vi "hmi_gun.vi"(11 "UserData":T1) -> ()   [LabVIEW 2011]
uses:
  user_data.ctl
  user_buttons_dualaction.ctl
  user_buttons_360.ctl
  gun/gun_tracking_mode.ctl
  signals/Signal.ctl
  Robot Global Data.vi
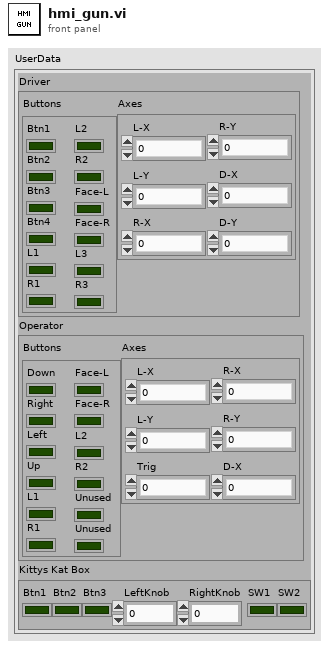
[diagram p1: front panel]
types:
  T1 = typedef "user_data.ctl" = cluster{"Driver":cluster{"Buttons":T2, "Axes":cluster{"L-X":dbl, "L-Y":dbl, "R-X":dbl, "R-Y":dbl, "D-X":dbl, "D-Y":dbl}}, "Operator":cluster{"Buttons":T3, "Axes":cluster{"L-X":dbl, "L-Y":dbl, "Trig":dbl, "R-X":dbl, "R-Y":dbl, "D-X":dbl}}, "Kittys Kat Box":cluster{"Btn1":bool, "Btn2":bool, "Btn3":bool, "LeftKnob":dbl, "RightKnob":dbl, "SW1":bool, "SW2":bool}}
  T2 = typedef "user_buttons_dualaction.ctl" = cluster{"Btn1":bool, "Btn2":bool, "Btn3":bool, "Btn4":bool, "L1":bool, "R1":bool, "L2":bool, "R2":bool, "Face-L":bool, "Face-R":bool, "L3":bool, "R3":bool}
  T3 = typedef "user_buttons_360.ctl" = cluster{"Down":bool, "Right":bool, "Left":bool, "Up":bool, "L1":bool, "R1":bool, "Face-L":bool, "Face-R":bool, "L2":bool, "R2":bool, "Unused":bool, "Unused":bool}
  T4 = typedef "gun_tracking_mode.ctl" = enum16{"manual_aim", "auto_aim_camera", "preset_center_field", "preset_right_pocket", "preset_left_pocket", "align_center", "align_center_backwards", "auto_aim_key", "align_fold", "auton_custom", "preset_pass", "auto_aim_auton"}
  T5 = typedef "Signal.ctl" = enum16{"SIGFIRE", "SIGSTOPSCRIPT", "SIGSTARTGUN", "SIGSTOPGUN", "SIGDISABLED", "SIGENABLED", "SIGUDPTIMEOUT", "SIGNEWVISION_REMOTE", "SIGNEWVISION_LOCAL", "SIGSHOTFIRED", "SIGDOTRACK", "SIGDONTTRACK"}
  T6 = enum16{"manual_aim", "auto_aim_camera", "preset_center_field", "preset_right_pocket", "preset_left_pocket"}
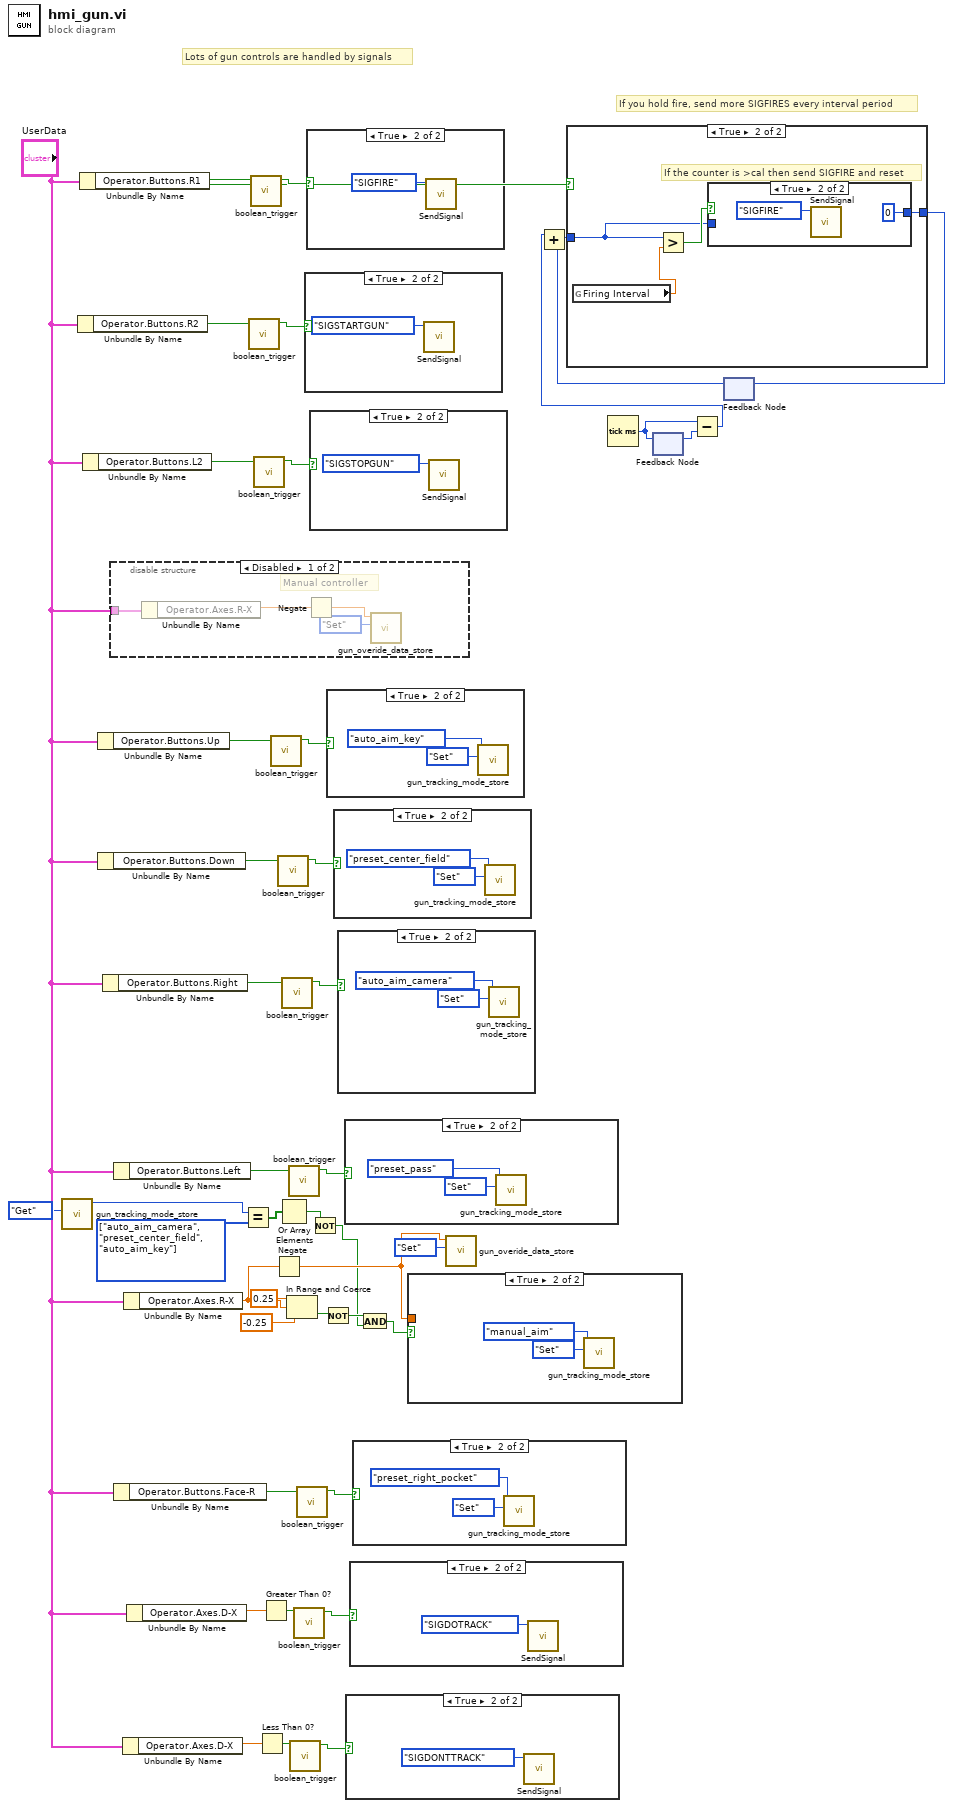
[diagram p0: block diagram]
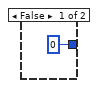
[diagram p7: hidden frame]
diagram:
  w7 = T4[] [enum."auto_aim_camera", enum."preset_center_field", enum."auto_aim_key"] items=["manual_aim", "auto_aim_camera", "preset_center_field", "preset_right_pocket", "preset_left_pocket", "align_center", "align_center_backwards", "auto_aim_key", "align_fold", "auton_custom", "preset_pass", "auto_aim_auton"]
  # "If you hold fire, send more SIGFIRES every interval period"
  # "Lots of gun controls are handled by signals"
  n1 = call "gun_tracking_mode_store.vi"("data_store_mode"=enum16{"Set", "Get"}."Get") -> ("gun tracking mode"=w8:T4)  [unwired: 10 in]
  n2 = Unbundle By Name("UserData") -> ("Operator.Buttons.R2"=w41:bool)
  n3 = Unbundle By Name("UserData") -> ("Operator.Buttons.R1"=w30:bool)
  n4 = Unbundle By Name("UserData") -> ("Operator.Buttons.L2"=w39:bool)
  n5 = Unbundle By Name("UserData") -> ("Operator.Buttons.Up"=w37:bool)
  n6 = Unbundle By Name("UserData") -> ("Operator.Buttons.Down"=w35:bool)
  n7 = Unbundle By Name("UserData") -> ("Operator.Buttons.Right"=w33:bool)
  n8 = disable-structure shown="Disabled" {
    disable-tunnel: "UserData" -> [w46 _]
    frame Disabled {
      # "Manual controller"
      n9 = Unbundle By Name(w46) -> ("Operator.Axes.R-X"=w44:dbl)
      n10 = Negate(x=w44) -> (-x=w45:dbl)
      n11 = call "gun_overide_data_store.vi"("mode"=enum16{"Set", "Get"}."Set", "Overide"=w45) -> ()  [unwired: 9 in, 1 out]
    }
    frame Enabled {
    }
  }
  n12 = Unbundle By Name("UserData") -> ("Operator.Buttons.Left"=w31:bool)
  n13 = Unbundle By Name("UserData") -> ("Operator.Buttons.Face-R"=w20:bool)
  n14 = Unbundle By Name("UserData") -> ("Operator.Axes.D-X"=w11:dbl)
  n15 = Unbundle By Name("UserData") -> ("Operator.Axes.R-X"=w19:dbl)
  n16 = Unbundle By Name("UserData") -> ("Operator.Axes.D-X"=w14:dbl)
  n17 = Equal?(x=w8, y=w7) -> (x = y?=w6:bool[])
  n18 = call "boolean_trigger.vi"("Input"=w41) -> ("Rising Edge"=w42:bool)  [unwired: 10 in]
  n19 = call "boolean_trigger.vi"("Input"=w30) -> ("Rising Edge"=w43:bool)  [unwired: 10 in]
  n20 = call "boolean_trigger.vi"("Input"=w39) -> ("Rising Edge"=w40:bool)  [unwired: 10 in]
  n21 = Less Than 0?(x=w11) -> (x < 0?=w12:bool)
  n22 = Greater Than 0?(x=w14) -> (x > 0?=w15:bool)
  n23 = call "boolean_trigger.vi"("Input"=w37) -> ("Rising Edge"=w38:bool)  [unwired: 10 in]
  n24 = Negate(x=w19) -> (-x=w17:dbl)
  n25 = call "boolean_trigger.vi"("Input"=w35) -> ("Rising Edge"=w36:bool)  [unwired: 10 in]
  n26 = Or Array Elements(Boolean array=w6) -> (logical OR=w2:bool)
  n27 = call "boolean_trigger.vi"("Input"=w33) -> ("Rising Edge"=w34:bool)  [unwired: 10 in]
  n28 = In Range and Coerce(upper limit=0.25, x=w19, lower limit=-0.25) -> (In Range?=w5:bool)  [unwired: 1 out]
  n29 = call "boolean_trigger.vi"("Input"=w31) -> ("Rising Edge"=w32:bool)  [unwired: 10 in]
  n30 = call "boolean_trigger.vi"("Input"=w12) -> ("Rising Edge"=w13:bool)  [unwired: 10 in]
  n31 = call "boolean_trigger.vi"("Input"=w15) -> ("Rising Edge"=w16:bool)  [unwired: 10 in]
  n32 = call "boolean_trigger.vi"("Input"=w20) -> ("Rising Edge"=w21:bool)  [unwired: 10 in]
  n33 = case shown="True" w42 {
    frame False {
    }
    frame True {
      n34 = call "SendSignal.vi"("Signal"=Signal."SIGSTARTGUN") -> ()  [unwired: 11 in]
    }
  }
  n35 = case shown="True" w43 {
    frame False {
    }
    frame True {
      n36 = call "SendSignal.vi"("Signal"=Signal."SIGFIRE") -> ()  [unwired: 11 in]
    }
  }
  n37 = case shown="True" w40 {
    frame False {
    }
    frame True {
      n38 = call "SendSignal.vi"("Signal"=Signal."SIGSTOPGUN") -> ()  [unwired: 11 in]
    }
  }
  n39 = Not(x=w2) -> (.not. x?=w1:bool)
  n40 = Not(x=w5) -> (.not. x?=w4:bool)
  n41 = case shown="True" w38 {
    frame False {
    }
    frame True {
      n42 = call "gun_tracking_mode_store.vi"("data_store_mode"=enum16{"Set", "Get"}."Set", "gun tracking mode"=gun_tracking_mode."auto_aim_key") -> ()  [unwired: 9 in, 1 out]
    }
  }
  n43 = case shown="True" w36 {
    frame False {
    }
    frame True {
      n44 = call "gun_tracking_mode_store.vi"("data_store_mode"=enum16{"Set", "Get"}."Set", "gun tracking mode"=gun_tracking_mode."preset_center_field") -> ()  [unwired: 9 in, 1 out]
    }
  }
  n45 = case shown="True" w34 {
    frame False {
    }
    frame True {
      n46 = call "gun_tracking_mode_store.vi"("data_store_mode"=enum16{"Set", "Get"}."Set", "gun tracking mode"=gun_tracking_mode."auto_aim_camera") -> ()  [unwired: 9 in, 1 out]
    }
  }
  n47 = case shown="True" w32 {
    frame False {
    }
    frame True {
      n48 = call "gun_tracking_mode_store.vi"("data_store_mode"=enum16{"Set", "Get"}."Set", "gun tracking mode"=gun_tracking_mode."preset_pass") -> ()  [unwired: 9 in, 1 out]
    }
  }
  n49 = case shown="True" w13 {
    frame False {
    }
    frame True {
      n50 = call "SendSignal.vi"("Signal"=Signal."SIGDONTTRACK") -> ()  [unwired: 11 in]
    }
  }
  n51 = case shown="True" w16 {
    frame False {
    }
    frame True {
      n52 = call "SendSignal.vi"("Signal"=Signal."SIGDOTRACK") -> ()  [unwired: 11 in]
    }
  }
  n53 = case shown="True" w21 {
    frame False {
    }
    frame True {
      n54 = call "gun_tracking_mode_store.vi"("data_store_mode"=enum16{"Set", "Get"}."Set", "gun tracking mode"=gun_tracking_mode."preset_right_pocket") -> ()  [unwired: 9 in, 1 out]
    }
  }
  n55 = And(x=w4, y=w1) -> (x .and. y?=w3:bool)
  n56 = case shown="True" w3 {
    tunnel: w17 -> [_ _]
    frame False {
    }
    frame True {
      n57 = call "gun_tracking_mode_store.vi"("data_store_mode"=enum16{"Set", "Get"}."Set", "gun tracking mode"=T6."manual_aim") -> ()  [unwired: 9 in, 1 out]
    }
  }
  n58 = call "gun_overide_data_store.vi"("mode"=enum16{"Set", "Get"}."Set", "Overide"=w17) -> ()  [unwired: 9 in, 1 out]
  n59 = Tick Count (ms)() -> (millisecond timer value=w29:u32)
  n60 = feedback-in #1(w29) -> ()
  n61 = feedback #1() -> (w28:u32)  [unwired: 1 in]
  n62 = Subtract(x=w29, y=w28) -> (x-y=w26:u32)
  n63 = feedback #2() -> (w27:u32)  [unwired: 1 in]
  n64 = Add(x=w26, y=w27) -> (x+y=w25:u32)
  n65 = case shown="True" w30 {
    tunnel: w25 -> [_ w68]
    tunnel: [u32 0 w67] -> w24
    frame False {
    }
    frame True {
      # "If the counter is >cal then send SIGFIRE and reset"
      n66 = global read "Robot Global Data.vi" "Firing Interval"() -> (w66:dbl)
      n67 = Greater?(x=w68, y=w66) -> (0:w69:bool)
      n68 = case shown="True" w69 {
        tunnel: w68 -> [w70 _]
        tunnel: [w70 u32 0] -> w67
        frame False {
        }
        frame True {
          n69 = call "SendSignal.vi"("Signal"=Signal."SIGFIRE") -> ()  [unwired: 11 in]
        }
      }
    }
  }
  n70 = feedback-in #2(w24) -> ()
